vi "get_unbinned.vi"() -> (0 "Counts per second":dbl, 1 "Counts":i32)   [LabVIEW 2013]
uses:
  phlib.dll
panel:
  out "iterations":i32
  out "Data":u32[](array[numeric]) format="%08x"
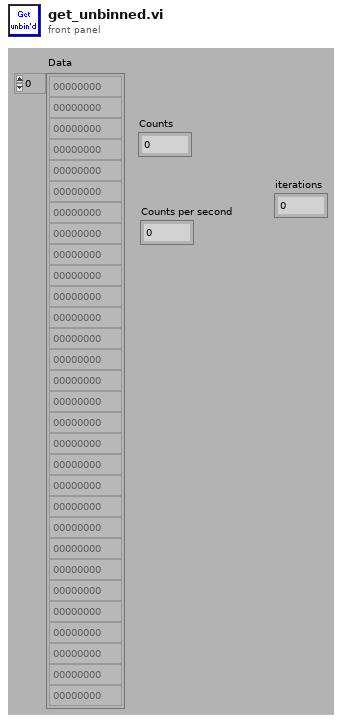
[diagram p1: front panel]
types:
  T1 = cluster{"Z_n":i32[], "devidx":i32, "initialized":bool, "acq time":i32, "Bin size":enum16{"1", "2", "4", "8", "16", "32", "64", "128"}, "# bins":i32, "sync rate":i32, "truncate":bool, "Ch0 Level":i32, "Ch1 Level":i32, "Ch0 ZeroX":i32, "Ch1 ZeroX":i32}
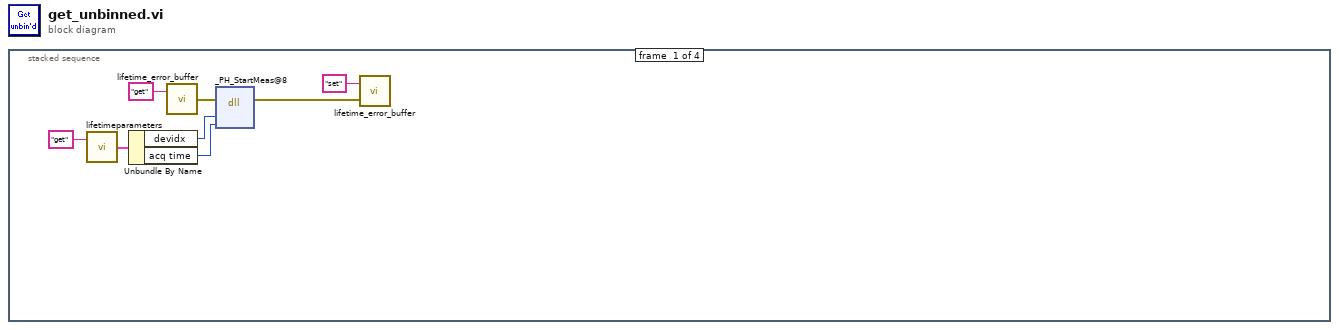
[diagram p0: block diagram]
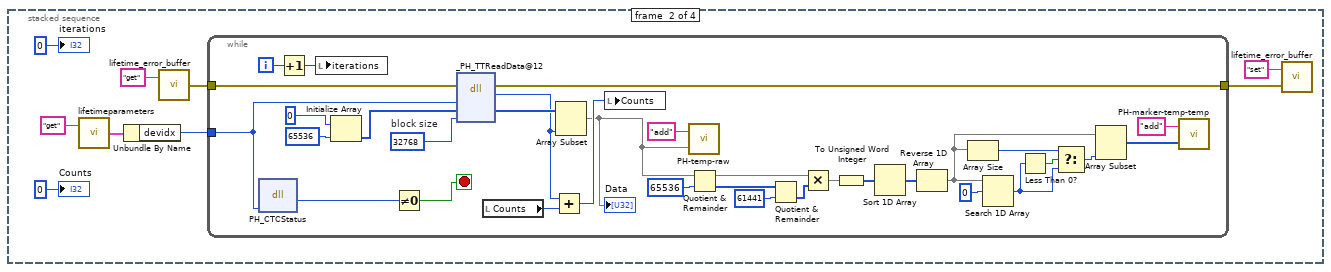
[diagram p2: hidden frame]
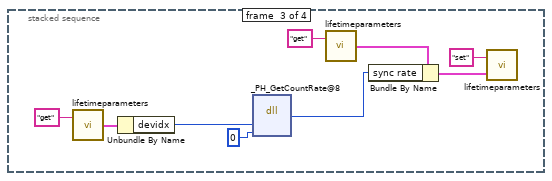
[diagram p3: hidden frame]
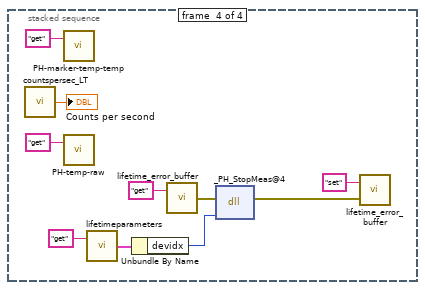
[diagram p4: hidden frame]
diagram:
  n1 = stacked-sequence {
    frame #0 {
      n2 = call "lifetimeparameters.vi"("command"="get") -> ("Params out"=w5:T1)  [unwired: 1 in]
      n3 = Unbundle By Name(w5) -> ("devidx"=w7:i32, "acq time"=w6:i32)
      n4 = call "lifetime_error_buffer.vi"("command"="get") -> ("error out"=w3:errorcluster)  [unwired: 1 in]
      n5 = dll-call lib="phlib.dll" fn="_PH_StartMeas@8" label="PH_StartMeas"(error in=w3, "devidx"=w7, "tacq"=w6) -> (error out=w1:errorcluster)  [unwired: 5 in, 1 out]
      n6 = call "lifetime_error_buffer.vi"("error in"=w1, "command"="set") -> ()  [unwired: 1 out]
    }
    frame #1 {
      n7 = call "lifetimeparameters.vi"("command"="get") -> ("Params out"=w12:T1)  [unwired: 1 in]
      n8 = Unbundle By Name(w12) -> ("devidx"=w11:i32)
      n9 = call "lifetime_error_buffer.vi"("command"="get") -> ("error out"=w16:errorcluster)  [unwired: 1 in]
      n10 = while {
        tunnel: w16 -> [w38]
        tunnel: [w37] -> w9
        tunnel: w11 -> [w18]
        i -> [w36]
        stop <- w46 stop-if-true
        w44 = 32768  # block size
        n11 = dll-call lib="phlib.dll" fn="PH_CTCStatus"("devidx"=w18) -> (w47:i32)  [unwired: 4 in, 2 out]
        n12 = Increment(x=w36) -> (x+1=w43:i32)
        n13 = local write "iterations"(w43) -> ()
        n14 = Initialize Array(u32 0, 65536) -> (w48:u32[])
        n15 = Not Equal To 0?(x=w47) -> (x != 0?=w46:bool)
        n16 = dll-call lib="phlib.dll" fn="_PH_TTReadData@12" label="PH_TTReadData"(error in=w38, "devidx"=w18, "buffer"=w48, "blocksize"=w44) -> (error out=w37:errorcluster, "return type"=w41:i32, "buffer"=w45:u32[])  [unwired: 4 in, 1 out]
        n17 = local read "Counts"() -> (w40:i32)
        n18 = Add(x=w41, y=w40) -> (x+y=w39:i32)
        n19 = Array Subset(array=w45, length=w41) -> (w33:u32[])  [unwired: 1 in]
        "Data" <- w33
        n20 = local write "Counts"(w39) -> ()
        n21 = call "PH-temp-raw.vi"("array in"=w33, "command"="add") -> ()  [unwired: 1 out]
        n22 = Quotient & Remainder(x=w33, y=u32 65536) -> (x-y*floor(x/y)=w19:u32[], floor(x/y)=w20:u32[])
        n23 = Quotient & Remainder(x=w20, y=u32 61441) -> (floor(x/y)=w22:u32[])  [unwired: 1 out]
        n24 = Multiply(x=w19, y=w22) -> (x*y=w30:u32[])
        n25 = To Unsigned Word Integer(number=w30) -> (unsigned 16bit integer=w21:u16[])
        n26 = Sort 1D Array(array=w21) -> (sorted array=w32:u16[])
        n27 = Reverse 1D Array(array=w32) -> (reversed array=w26:u16[])
        n28 = Array Size(array=w26) -> (size(s)=w25:i32)
        n29 = Search 1D Array(1D array=w26, element=u16 0) -> (index of element=w27:i32)  [unwired: 1 in]
        n30 = Less Than 0?(x=w27) -> (x < 0?=w28:bool)
        n31 = Select(t=w25, s=w28, f=w27) -> (s? t:f=w24:i32)
        n32 = Array Subset(array=w26, length=w24) -> (w29:u16[])  [unwired: 1 in]
        n33 = call "PH-marker-temp-temp.vi"("array in"=w29, "command"="add") -> ()  [unwired: 1 out]
      }
      n34 = call "lifetime_error_buffer.vi"("error in"=w9, "command"="set") -> ()  [unwired: 1 out]
      "iterations" <- 0 ("iterations")
      "Counts" <- 0 ("iterations")
    }
    frame #2 {
      n35 = call "lifetimeparameters.vi"("command"="get") -> ("Params out"=w52:T1)  [unwired: 1 in]
      n36 = Unbundle By Name(w52) -> ("devidx"=w51:i32)
      n37 = dll-call lib="phlib.dll" fn="_PH_GetCountRate@8" label="PH_GetCountRate"("devidx"=w51, "channel"=0) -> (w54:i32)  [unwired: 5 in, 2 out]
      n38 = call "lifetimeparameters.vi"("command"="get") -> ("Params out"=w56:T1)  [unwired: 1 in]
      n39 = Bundle By Name(cluster=w56, "sync rate"=w54) -> (w55:T1)
      n40 = call "lifetimeparameters.vi"("Params in"=w55, "command"="set") -> ()  [unwired: 1 out]
    }
    frame #3 {
      n41 = call "countspersec_LT.vi"() -> ("Avg cts/s"=→"Counts per second":dbl)
      n42 = call "PH-marker-temp-temp.vi"("command"="get") -> ()  [unwired: 1 in, 1 out]
      n43 = call "PH-temp-raw.vi"("command"="get") -> ()  [unwired: 1 in, 1 out]
      n44 = call "lifetimeparameters.vi"("command"="get") -> ("Params out"=w63:T1)  [unwired: 1 in]
      n45 = Unbundle By Name(w63) -> ("devidx"=w62:i32)
      n46 = call "lifetime_error_buffer.vi"("command"="get") -> ("error out"=w60:errorcluster)  [unwired: 1 in]
      n47 = dll-call lib="phlib.dll" fn="_PH_StopMeas@4" label="PH_StopMeas"(error in=w60, "devidx"=w62) -> (error out=w68:errorcluster)  [unwired: 4 in, 1 out]
      n48 = call "lifetime_error_buffer.vi"("error in"=w68, "command"="set") -> ()  [unwired: 1 out]
    }
  }
